vi "Drive_Utils_DistanceRadiusToLeftRight.vi"(3 "error in":errorcluster, 4 "Turn Radius":dbl, 5 "Distance":dbl) -> (0 "error out":errorcluster, 1 "Right Distance":dbl, 2 "Left Distance":dbl)   [LabVIEW 2009, in "Drive.lvlib" / "Drive_Utils.lvlib"]
uses:
  Drive_Utils.lvlib
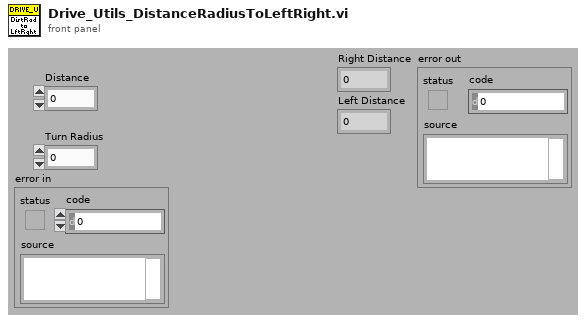
[diagram p1: front panel]
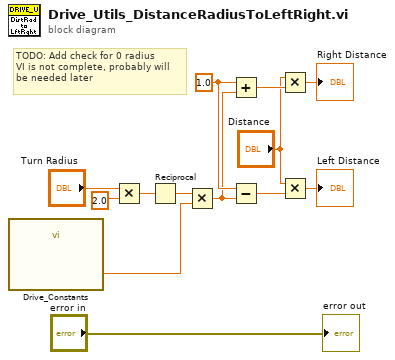
[diagram p0: block diagram]
diagram:
  w7 = 1.0 ("y")
  # "TODO: Add check for 0 radius\nVI is not complete, probably will\nbe needed later"
  n1 = call "Drive_Constants.vi"() -> ("Wheels interval (m)"=w1:dbl)  [unwired: 23 in, 4 out]
  n2 = Multiply(x="Turn Radius", y=2.0) -> (x*y=w11:dbl)
  n3 = Reciprocal(x=w11) -> (1/x=w10:dbl)
  n4 = Multiply(x=w10, y=w1) -> (x*y=w6:dbl)
  n5 = Add(x=w7, y=w6) -> (x+y=w9:dbl)
  n6 = Subtract(x=w7, y=w6) -> (x-y=w4:dbl)
  n7 = Multiply(x="Distance", y=w9) -> (x*y=→"Right Distance":dbl)
  n8 = Multiply(x="Distance", y=w4) -> (x*y=→"Left Distance":dbl)
  "error out" <- "error in"
